vi "PH_Beckhoff.evt Call Set Boolean Value.vi"(0 "i ref in":refnum<vi>, 2 "Beckhoff Instance":string, 3 "Tagname to set":string, 4 "Value":bool, 5 "error in":errorcluster) -> (14 "i ref out":refnum<vi>, 19 "error out":errorcluster)   [LabVIEW 2014, in "PH_Beckhoff.lvlib"]
uses:
  PH_Beckhoff.lvlib
  CS_Core/CSSystem/CoreLib/CoreLib.string 2 byte array.vi
  CS_Core/CSSystem/CoreLib/CoreLib.short 2 byte array.vi
  CS_Core/BaseProcess/BaseProcess.lvlib
  CS_Core/CSSystem/CoreLib/CoreLib.lvlib
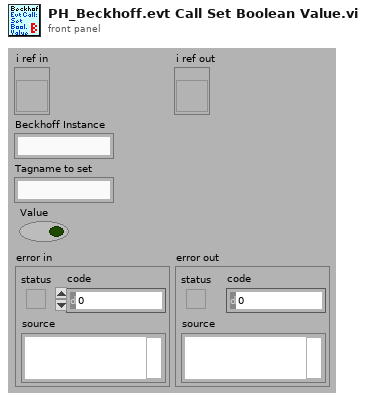
[diagram p1: front panel]
types:
  T1 = typedef "CoreDefs.rawDataType.ctl" = i8[]
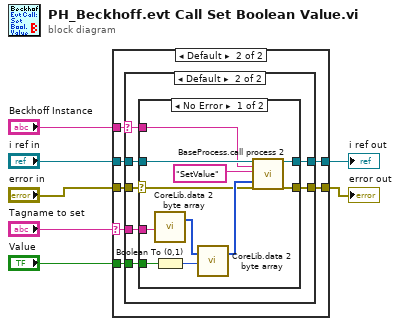
[diagram p0: block diagram]
diagram:
  n1 = case shown="Default" "Tagname to set" {
    selector: "Tagname to set" -> [_ w10]
    tunnel: "error in" -> [w8 w16]
    tunnel: "Value" -> [_ w15]
    tunnel: [w9 w14] -> w5
    tunnel: "i ref in" -> [w9 w13]
    tunnel: [w8 w12] -> w3
    tunnel: "Beckhoff Instance" -> [_ w11]
    frame "", "N/A" {
    }
    frame Default {
      n2 = case shown="Default" w11 {
        selector: w11 -> [_ w19]
        tunnel: w16 -> [w17 w25]
        tunnel: w15 -> [_ w24]
        tunnel: w10 -> [_ w23]
        tunnel: [w18 w22] -> w14
        tunnel: w13 -> [w18 w21]
        tunnel: [w17 w20] -> w12
        frame "", "N/A" {
        }
        frame Default {
          n3 = case shown="No Error" w25 {
            selector: w25 -> [w26 w37]
            tunnel: [w36 w37] -> w20
            tunnel: w21 -> [w35 w38]
            tunnel: [w34 w38] -> w22
            tunnel: w19 -> [w33 _]
            tunnel: w23 -> [w29 _]
            tunnel: w24 -> [w28 _]
            frame No Error {
              n4 = call-poly "CoreLib.data 2 byte array.vi"("string"=w29) -> ("byteArray out"=w31:T1)  [unwired: 18 in]
              n5 = Boolean To (0,1)(Boolean=w28) -> (0, 1=w27:i16)
              n6 = call-poly "CoreLib.data 2 byte array.vi"("byteArray"=w31, "i16"=w27) -> ("byteArray out"=w30:T1)  [unwired: 17 in]
              n7 = call "BaseProcess.call process 2.vi"("i ref in"=w35, "Object"=w33, "Selector"="SetValue", "Data"=w30, "error in (no error)"=w26) -> ("i ref out"=w34:refnum<vi>, "error out"=w36:errorcluster)  [unwired: 13 in]
            }
            frame Error {
            }
          }
        }
      }
    }
  }
  "i ref out" <- w5
  "error out" <- w3
